vi "Dequeue Open Report.vi"(8 "error in (no error)":errorcluster, 9 "timeout in ms (0)":i32, 11 "Mock Report In":refnum<class "Mock Report.lvclass">) -> (0 "error out":errorcluster, 1 "timed out?":bool, 2 "path":path, 3 "Mock Report Out":refnum<class "Mock Report.lvclass">)   [LabVIEW 2020, in "Mock Report.lvclass"]
uses:
  Mock Report.lvclass
  Mock Report.lvclass/Mock Report.ctl
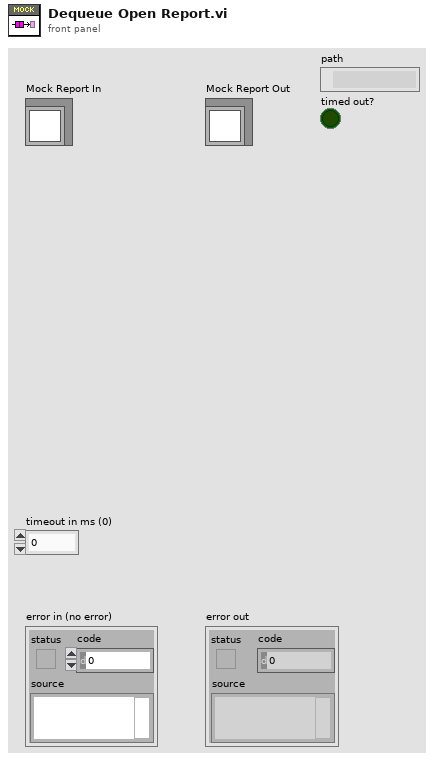
[diagram p1: front panel]
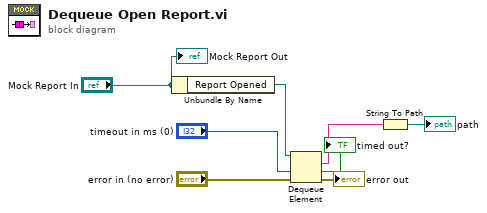
[diagram p0: block diagram]
diagram:
  n1 = Unbundle By Name("Mock Report In") -> ("Report Opened"=w4:refnum<queue>)
  n2 = Dequeue Element(queue=w4, timeout in ms (-1)="timeout in ms (0)", error in (no error)="error in (no error)") -> (element=w3:string, timed out?=→"timed out?":bool, error out=→"error out":errorcluster)  [unwired: 1 out]
  n3 = String To Path(string=w3) -> (path=→"path":path)
  "Mock Report Out" <- "Mock Report In"
